vi "LCD Reset.vi"(8 "error in":errorcluster, 11 "FPGA VI Reference Out 2":refnum<k20>) -> (0 "error out":errorcluster, 3 "FPGA VI Reference Out":refnum<k20>)   [LabVIEW 2019]
uses:
  <vilib>/Utility/error.llb/Error Cluster From Error Code.vi
  <vilib>/rvi/errors/niLvFpgaAdjustHostInterfaceError.vi
  <vilib>/rvi/interface/nirviMethod/nirviMethod.xnode
  <vilib>/FPGAPlugInAG/Dynamic/niLvFpga_WriteFifo_Dynamic.vi
  <vilib>/rvi/errors/niLvFpgaMergeErrorWithErrorCode.vi
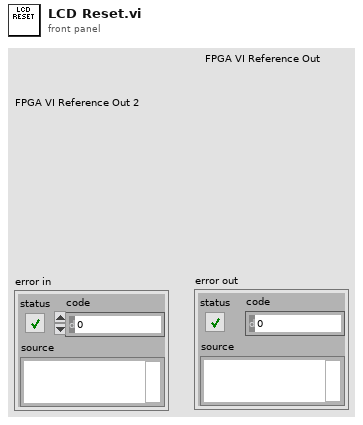
[diagram p1: front panel]
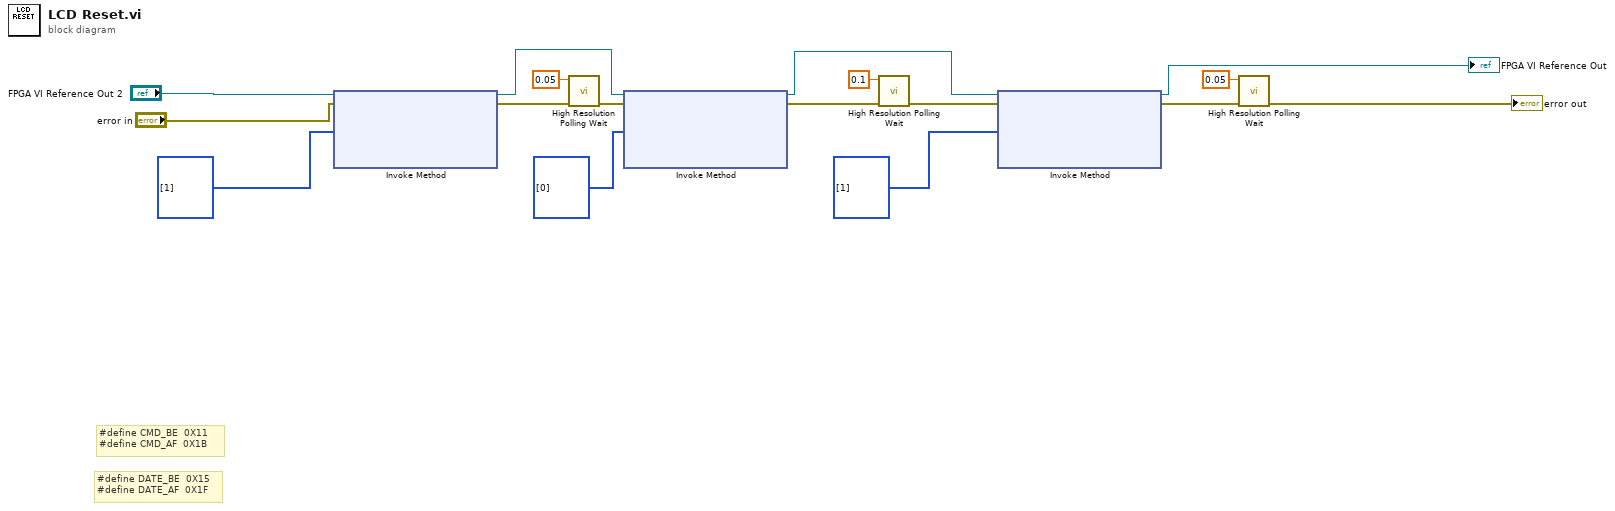
[diagram p0: block diagram]
diagram:
  # "#define DATE_BE\t\t0X15\n#define DATE_AF\t\t0X1F"
  # "#define CMD_BE\t\t0X11\n#define CMD_AF\t\t0X1B"
  n1 = xnode "Invoke Method"("FPGA VI Reference In"="FPGA VI Reference Out 2", "error in"="error in", "Data"=u64[] [1]) -> ("FPGA VI Reference Out"=w16:refnum<k20>, "error out"=w17:errorcluster)  [unwired: 1 in, 1 out]
  n2 = call <vilib>:"High Resolution Polling Wait.vi"("error in (no error)"=w17, "seconds to wait"=0.05) -> ("error out"=w15:errorcluster)  [unwired: 9 in]
  n3 = xnode "Invoke Method"("FPGA VI Reference In"=w16, "error in"=w15, "Data"=u64[] [0]) -> ("FPGA VI Reference Out"=w7:refnum<k20>, "error out"=w9:errorcluster)  [unwired: 1 in, 1 out]
  n4 = call <vilib>:"High Resolution Polling Wait.vi"("error in (no error)"=w9, "seconds to wait"=0.1) -> ("error out"=w8:errorcluster)  [unwired: 9 in]
  n5 = xnode "Invoke Method"("FPGA VI Reference In"=w7, "error in"=w8, "Data"=u64[] [1]) -> ("FPGA VI Reference Out"=→"FPGA VI Reference Out":refnum<k20>, "error out"=w4:errorcluster)  [unwired: 1 in, 1 out]
  n6 = call <vilib>:"High Resolution Polling Wait.vi"("error in (no error)"=w4, "seconds to wait"=0.05) -> ("error out"=→"error out":errorcluster)  [unwired: 9 in]
